vi "LoadCounterCfg.vi"() -> (3 "Variant":variant)   [LabVIEW 2012, in "NEVSTOP QD Shortcuts.lvlib"]
uses:
  NEVSTOP QD Shortcuts.lvlib
  <userlib>/_OpenG.lib/string/string.llb/Trim Whitespace (String Array)__ogtk.vi
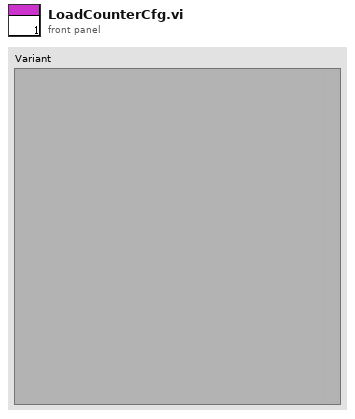
[diagram p1: front panel]
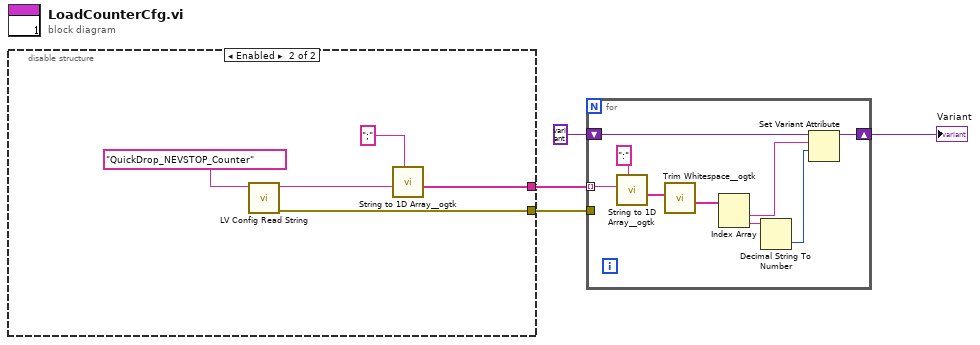
[diagram p0: block diagram]
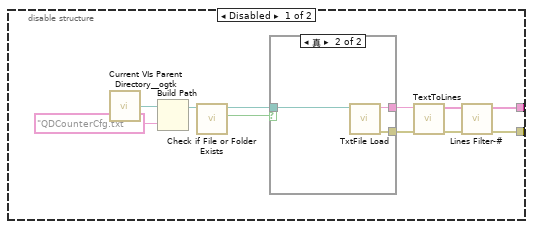
[diagram p2: hidden frame]
diagram:
  n1 = disable-structure shown="Enabled" {
    disable-tunnel: [w7 w19] -> w3
    disable-tunnel: [w6 w22] -> w2
    frame Disabled {
      n2 = call <userlib>:"Current VIs Parent Directory__ogtk.vi"() -> ("Parent Directory (+ Relative)"=w12:path)  [unwired: 5 in]
      n3 = Build Path(base path=w12, name or relative path="QDCounterCfg.txt") -> (appended path=w13:path)
      n4 = call <vilib>:"Check if File or Folder Exists.vi"("path"=w13) -> ("file or folder exists?"=w5:bool, "dup path"=w15:path)  [unwired: 8 in, 1 out]
      n5 = case shown="真" w5 {
        tunnel: w15 -> [_ w18]
        tunnel: [_ w17] -> w11
        tunnel: [_ w16] -> w10
        frame False {
        }
        frame True {
          n6 = call "TxtFile Load.vi"("Path"=w18) -> ("error out"=w17:errorcluster, "text"=w16:string)  [unwired: 9 in]
        }
      }
      n7 = call "TextToLines.vi"("error in (no error)"=w11, "string"=w10) -> ("error out"=w9:errorcluster, "Lines"=w8:string[])  [unwired: 8 in]
      n8 = call "Lines Filter-#.vi"("error in (no error)"=w9, "Lines"=w8) -> ("error out"=w6:errorcluster, "Config Text List"=w7:string[])  [unwired: 8 in]
    }
    frame Enabled {
      n9 = call <resource>:"LV Config Read String.vi"("key"="QuickDrop_NEVSTOP_Counter") -> ("error out"=w22:errorcluster, "value"=w21:string)  [unwired: 4 in, 1 out]
      n10 = call <userlib>:"String to 1D Array__ogtk.vi"("delimiter (Tab)"=";", "string"=w21) -> ("Array of Strings"=w19:string[])  [unwired: 9 in]
    }
  }
  n11 = for {
    tunnel: w3 -> [w32] mode=indexing
    tunnel: w2 -> [_]
    shift-right: [w29] -> w4
    shift-left: variant ("Variant") -> [w28]
    n12 = call <userlib>:"String to 1D Array__ogtk.vi"("delimiter (Tab)"=":", "string"=w32) -> ("Array of Strings"=w30:string[])  [unwired: 9 in]
    n13 = call-poly <userlib>:"Trim Whitespace__ogtk.vi"("String in"=w30) -> ("String out"=w27:string[])  [unwired: 6 in]
    n14 = Index Array(array=w27) -> (element #1=w26:string, element #2=w25:string)  [unwired: 2 in]
    n15 = Decimal String To Number(string=w25) -> (number=w24:i32)  [unwired: 2 in, 1 out]
    n16 = Set Variant Attribute(Variant=w28, name=w26, value=w24) -> (Variant out=w29:variant)  [unwired: 1 in, 2 out]
  }
  "Variant" <- w4
